vi "Static training image.vi"(1 "Image in":T1, 2 "Training image on/off":bool) -> (0 "Image out":T1)   [LabVIEW 2022 SP3]
doc: "Allows for testing of the computer vision without camera in the rigth position\nIf input = false -> Input image is just passed trough\nIf input = true -> Training image is loaded and exported"
uses:
  <vilib>/vision/Image Controls.llb/IMAQ Image.ctl
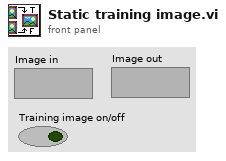
[diagram p1: front panel]
types:
  T1 = typedef "IMAQ Image.ctl" = refnum<image>
  T2 = typedef "imagedata.ctl" = cluster{"image type":i32, "image depth":i32, "image":u8[], "mask":u8[], "colors":u32[], "Rectangle":cluster{"left":i16, "top":i16, "right":i16, "bottom":i16}}
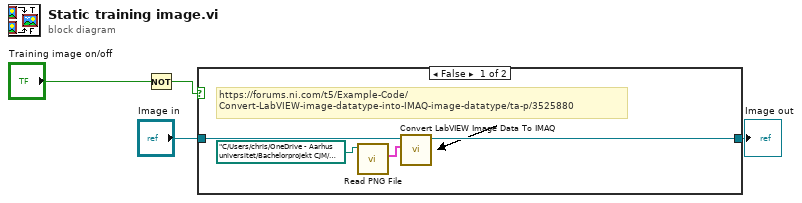
[diagram p0: block diagram]
diagram:
  n1 = Not(x="Training image on/off") -> (.not. x?=w1:bool)
  n2 = case shown="False" w1 {
    tunnel: "Image in" -> [w6 w9]
    tunnel: [w5 w9] -> w3
    frame False {
      # "https://forums.ni.com/t5/Example-Code/\nConvert-LabVIEW-image-datatype-into-IMAQ-image-datatype/ta-p/3525880"
      n3 = call <vilib>:"Read PNG File.vi"("path to PNG file"=path "C:/Users/chris/OneDrive - Aarhus universitet/Bachelorprojekt CJM/Kode/CV/tempbillede.png") -> ("image data"=w8:T2)  [unwired: 8 in, 2 out]
      n4 = call "Convert LabVIEW Image Data To IMAQ.vi"("Image Data"=w8, "Image In"=w6) -> ("Image Out"=w5:T1)  [unwired: 8 in, 1 out]
    }
    frame True {
    }
  }
  "Image out" <- w3
